vi "Test - Restartable.vi"() -> ()   [LabVIEW 2018]
uses:
  Ammeter.ctl
  <vilib>/DAQmx/read.llb/DAQmx Read (Analog 1D Wfm NChan NSamp).vi
  <vilib>/DAQmx/create/channels.llb/DAQmx Create Channel (AI-Voltage-Basic).vi
  <vilib>/DAQmx/create/channels.llb/DAQmx Create Channel (CI-Pulse Ticks).vi
  <vilib>/DAQmx/miscellaneous.llb/DAQmx Fill In Error Info.vi
panel:
  in  "?":enum32{"Monitor", "Calibration", "Future Use"}(tab)
  out "GPMDischarge":T1 caption="Dis GPM" format="%2.0f"
  out "GPMCase":T1 caption="Case GPM" format="%2.0f"
  out "PSI Case":T1 caption="Case PSI" format="%2.0f"
  out "PSI In":T1 caption="Inlet PSI" format="%2.0f"
  out "PSI Discharge":T1 caption="Dis PSI" format="%2.0f"
  out "Amps C":dbl format="%#.2g"
  out "Amps B":dbl format="%#.2g"
  out "Amps A":dbl format="%#.2g"
  out "VAC C":dbl caption="Vac" format="%#_3f"
  out "VAC B":dbl caption="Vac" format="%#_3f"
  out "VAC A":dbl caption="Vac" format="%#_3f"
  out "AC Hz":dbl caption="Hz" format="%#_3f"
  in  "Stop Button":bool
  in  "Loop Delay":u32=5
  out "Waveform Chart":waveform(dbl)[](graph)
  in  "Stop Button 2":bool
  in  "Boolean":bool
  in  "CaseGPM Offset":dbl format="%#_13g"
  in  "CaseGPM Scale":dbl=1.0 format="%#_13g"
  out "CaseGPM":dbl caption="Indicated"
  in  "DisGPM Offset":dbl format="%#_13g"
  in  "DisGPM Scale":dbl=1.0 format="%#_13g"
  out "DisGPM":dbl caption="Indicated"
  in  "CasePSI Offset":dbl format="%#_13g"
  in  "CasePSI Scale":dbl=200.0 format="%#_13g"
  out "CasePSI":dbl caption="Indicated"
  in  "InPSI Offset":dbl format="%#_13g"
  in  "InPSI Scale":dbl=100.0 format="%#_13g"
  out "InPSI Ind":dbl caption="Indicated"
  in  "DisPSI Offset":dbl format="%#_13g"
  in  "DisPSI Scale":dbl=1000.0 format="%#_13g"
  out "DisPSI Ind":dbl caption="Indicated"
  out "AC Freq Ind":dbl caption="Indicated"
  in  "AC Freq Offset":dbl=10.0 caption="Offset" format="%#_13g"
  in  "AC Freq Scale":dbl=100.0 caption="Scale" format="%#_13g"
  out "A VAC Ind":dbl caption="Indicated"
  in  "VAC Offset A":dbl caption="Offset" format="%#_13g"
  in  "VAC Scale A":dbl=50.0 caption="Scale" format="%#_13g"
  out "B VAC Ind":dbl caption="Indicated"
  in  "Amp Offset C":dbl format="%#_13g"
  in  "Amp Offset B":dbl format="%#_13g"
  in  "Amp Offset A":dbl format="%#_13g"
  in  "Amp Scale C":dbl=9.88 format="%#_13g"
  in  "Amp Scale B":dbl=9.88 format="%#_13g"
  in  "Amp Scale A":dbl=9.88 format="%#_13g"
  in  "VAC Scale B":dbl=50.0 caption="Scale" format="%#_13g"
  in  "VAC Offset B":dbl caption="Offset" format="%#_13g"
  in  "VAC Offset C":dbl caption="Offset" format="%#_13g"
  in  "VAC Scale C":dbl=50.0 caption="Scale" format="%#_13g"
  out "C VAC Ind":dbl caption="Indicated"
  out "A VAmp Ind":dbl caption="Indicated"
  out "B VAmp Ind":dbl caption="Indicated"
  out "C VAmp Ind":dbl caption="Indicated"
  out "error out":errorcluster
  # "AC Frequency"
  # "A Phase VAC"
  # "B Phase VAC"
  # "C Phase VAC"
  # "A Phase Amps"
  # "B Phase Amps"
  # "C Phase Amps"
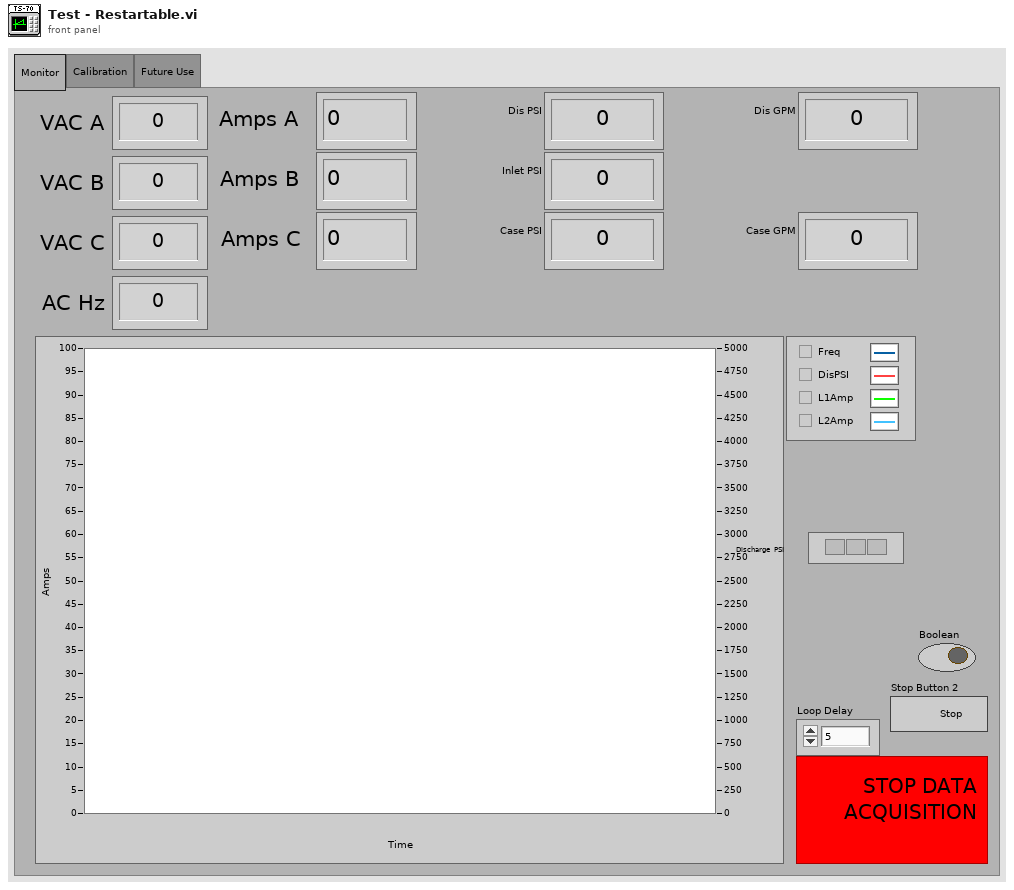
[diagram p1: front panel]
types:
  T1 = typedef "Ammeter.ctl" = dbl
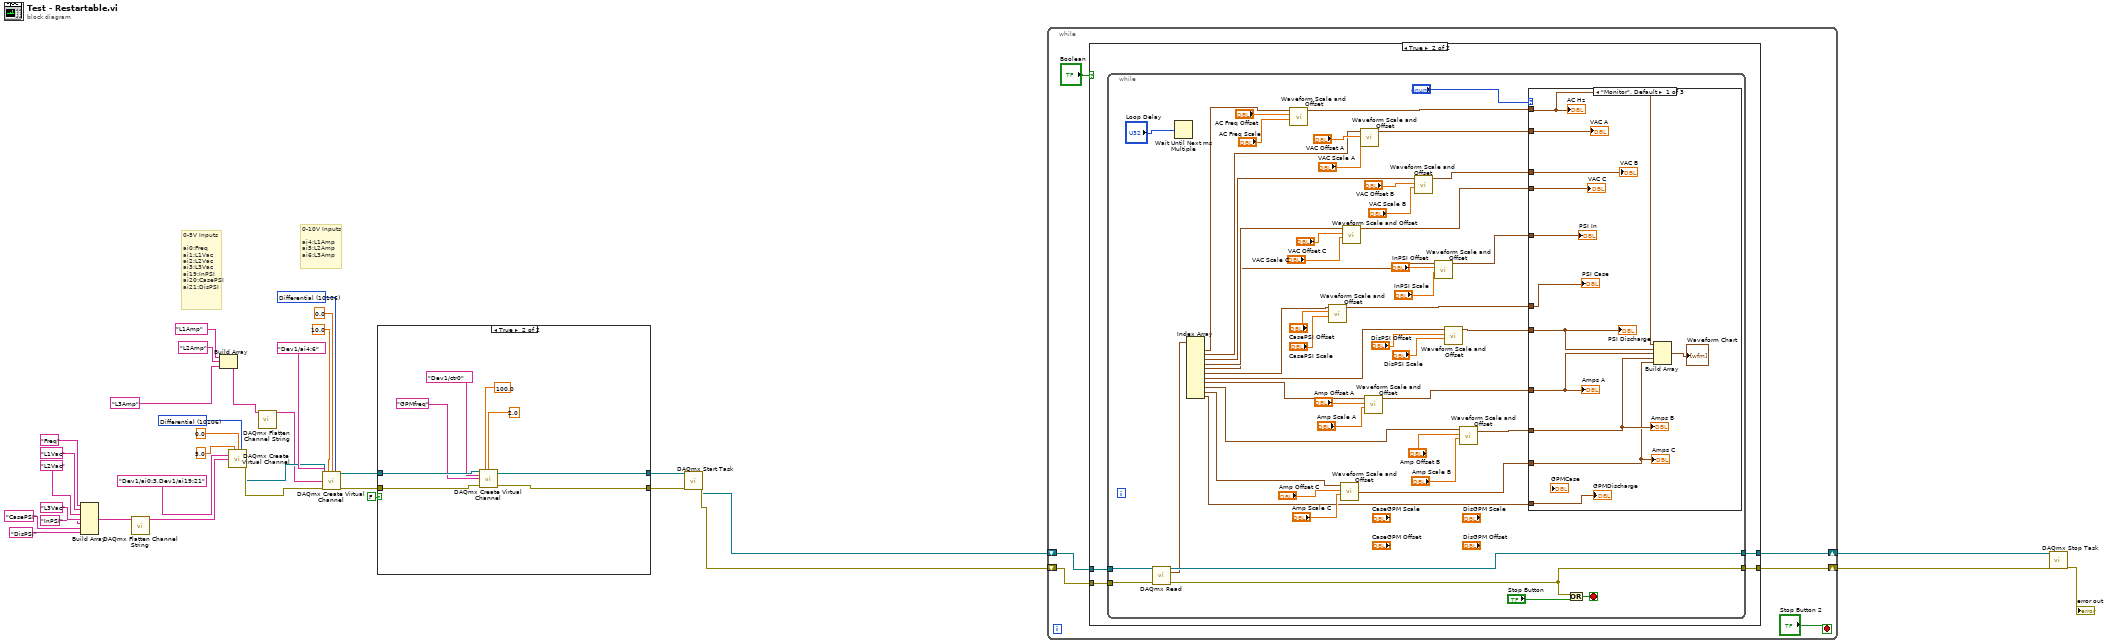
[diagram p0: block diagram]
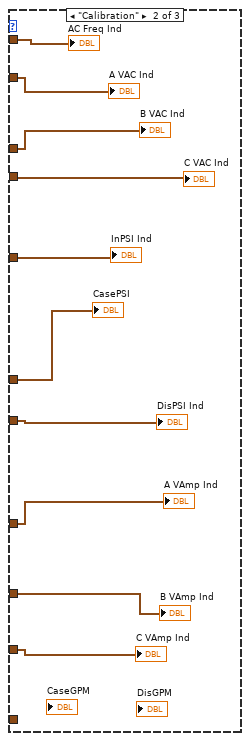
[diagram p4: hidden frame]
diagram:
  w28 = 10106 items=["default"=-1, "RSE"=10083, "NRSE"=10078, "Differential"=10106, "Pseudodifferential"=12529] ("input terminal configuration")
  w31 = 10106 items=["default"=-1, "RSE"=10083, "NRSE"=10078, "Differential"=10106, "Pseudodifferential"=12529] ("input terminal configuration")
  # "0-10V Inputs\n\nai4:L1Amp\nai5:L2Amp\nai6:L3Amp"
  # "0-5V Inputs\n\nai0:Freq\nai1:L1Vac\nai2:L2Vac\nai3:L3Vac\nai19:InPSI\nai20:CasePSI\nai21:DisPSI"
  n1 = Build Array("Freq", "L1Vac", "L2Vac", "L3Vac", "InPSI" ("element"), "CasePSI", "DisPSI") -> (w14:string[])
  n2 = call <vilib>:"DAQmx Flatten Channel String.vi"("names in"=w14) -> ("names out"=w13:string)  [unwired: 13 in, 1 out]
  n3 = Build Array("L1Amp", "L2Amp", "L3Amp") -> (w11:string[])
  n4 = call-poly <vilib>:"DAQmx Create Virtual Channel.vi"("maximum value"=5.0, "minimum value"=0.0, "input terminal configuration"=w31, "physical channels"=tag "Dev1/ai0:3,Dev1/ai19:21", "name to assign"=w13) -> ("task out"=w24:refnum<k21>, "error out"=w25:errorcluster)  [unwired: 9 in]
  n5 = call <vilib>:"DAQmx Flatten Channel String.vi"("names in"=w11) -> ("names out"=w7:string)  [unwired: 13 in, 1 out]
  n6 = call-poly <vilib>:"DAQmx Create Virtual Channel.vi"("task in"=w24, "maximum value"=10.0, "minimum value"=0.0, "input terminal configuration"=w28, "physical channels"=tag "Dev1/ai4:6", "name to assign"=w7, "error in"=w25) -> ("task out"=w5:refnum<k21>, "error out"=w3:errorcluster)  [unwired: 7 in]
  n7 = case shown="True" FALSE {
    tunnel: w5 -> [w36 w44]
    tunnel: [w36 w43] -> w4
    tunnel: w3 -> [w35 w42]
    tunnel: [w35 w41] -> w2
    frame False {
    }
    frame True {
      n8 = call-poly <vilib>:"DAQmx Create Virtual Channel.vi"("task in"=w44, "maximum value"=100.0, "minimum value"=2.0, "counter"=tag "Dev1/ctr0", "name to assign"="GPMfreq", "error in"=w42) -> ("task out"=w43:refnum<k21>, "error out"=w41:errorcluster)  [unwired: 8 in]
    }
  }
  n9 = call <vilib>:"DAQmx Start Task.vi"("task/channels in"=w4, "error in"=w2) -> ("task out"=w6:refnum<k21>, "error out"=w34:errorcluster)  [unwired: 12 in]
  n10 = while {
    shift-right: [w49] -> w23
    shift-left: w34 -> [w50]
    shift-right: [w48] -> w22
    shift-left: w6 -> [w47]
    stop <- "Stop Button 2" stop-if-true
    n11 = case shown="True" "Boolean" {
      tunnel: w50 -> [w51 w56]
      tunnel: [w51 w55] -> w49
      tunnel: [w52 w54] -> w48
      tunnel: w47 -> [w52 w53]
      frame False {
      }
      frame True {
        n12 = while {
          tunnel: w53 -> [w106]
          tunnel: w56 -> [w105]
          tunnel: [w101] -> w55
          tunnel: [w100] -> w54
          stop <- w102 stop-if-true
          n13 = call-poly <vilib>:"DAQmx Read.vi"("task/channels in"=w106, "error in"=w105) -> ("task out"=w100:refnum<k21>, "data"=w87:waveform(dbl)[], "error out"=w101:errorcluster)  [unwired: 11 in]
          n14 = Wait Until Next ms Multiple(millisecond multiple="Loop Delay") -> ()  [unwired: 1 out]
          n15 = Index Array(array=w87) -> (element #1=w72:waveform(dbl), element #2=w88:waveform(dbl), element #3=w82:waveform(dbl), element #4=w81:waveform(dbl), element #5=w64:waveform(dbl), element #6=w59:waveform(dbl), element #7=w68:waveform(dbl), element #8=w97:waveform(dbl), element #9=w92:waveform(dbl), element #10=w91:waveform(dbl), element #11=w57:waveform(dbl))  [unwired: 11 in]
          n16 = call <vilib>:"Waveform Scale and Offset.vi"("scale"="AC Freq Scale", "offset"="AC Freq Offset", "waveform in"=w72) -> ("waveform out"=w73:waveform(dbl))  [unwired: 7 in, 1 out]
          n17 = call <vilib>:"Waveform Scale and Offset.vi"("scale"="CasePSI Scale", "offset"="CasePSI Offset", "waveform in"=w59) -> ("waveform out"=w58:waveform(dbl))  [unwired: 7 in, 1 out]
          n18 = call <vilib>:"Waveform Scale and Offset.vi"("scale"="Amp Scale C", "offset"="Amp Offset C", "waveform in"=w91) -> ("waveform out"=w71:waveform(dbl))  [unwired: 7 in, 1 out]
          n19 = call <vilib>:"Waveform Scale and Offset.vi"("scale"="VAC Scale C", "offset"="VAC Offset C", "waveform in"=w81) -> ("waveform out"=w77:waveform(dbl))  [unwired: 7 in, 1 out]
          n20 = call <vilib>:"Waveform Scale and Offset.vi"("scale"="VAC Scale A", "offset"="VAC Offset A", "waveform in"=w88) -> ("waveform out"=w79:waveform(dbl))  [unwired: 7 in, 1 out]
          n21 = call <vilib>:"Waveform Scale and Offset.vi"("scale"="Amp Scale A", "offset"="Amp Offset A", "waveform in"=w97) -> ("waveform out"=w70:waveform(dbl))  [unwired: 7 in, 1 out]
          n22 = call <vilib>:"Waveform Scale and Offset.vi"("scale"="VAC Scale B", "offset"="VAC Offset B", "waveform in"=w82) -> ("waveform out"=w78:waveform(dbl))  [unwired: 7 in, 1 out]
          n23 = call <vilib>:"Waveform Scale and Offset.vi"("scale"="InPSI Scale", "offset"="InPSI Offset", "waveform in"=w64) -> ("waveform out"=w65:waveform(dbl))  [unwired: 7 in, 1 out]
          n24 = call <vilib>:"Waveform Scale and Offset.vi"("scale"="DisPSI Scale", "offset"="DisPSI Offset", "waveform in"=w68) -> ("waveform out"=w69:waveform(dbl))  [unwired: 7 in, 1 out]
          n25 = call <vilib>:"Waveform Scale and Offset.vi"("scale"="Amp Scale B", "offset"="Amp Offset B", "waveform in"=w92) -> ("waveform out"=w76:waveform(dbl))  [unwired: 7 in, 1 out]
          n26 = case shown="\"Monitor\", Default" "?" {
            tunnel: w79 -> [w118 w128 _]
            tunnel: w78 -> [w117 w126 _]
            tunnel: w77 -> [w116 w125 _]
            tunnel: w76 -> [w110 w124 _]
            tunnel: w71 -> [w109 w121 _]
            tunnel: w73 -> [w108 w127 _]
            tunnel: w70 -> [w115 w123 _]
            tunnel: w69 -> [w114 w122 _]
            tunnel: w65 -> [w112 w120 _]
            tunnel: w58 -> [w111 w119 _]
            tunnel: w57 -> [w107 _ _]
            frame "Monitor", Default {
              n27 = Build Array(w108, w114, w115, w110, w109) -> (→"Waveform Chart":waveform(dbl)[])
              "VAC A" <- w118
              "VAC B" <- w117
              "VAC C" <- w116
              "Amps B" <- w110
              "Amps C" <- w109
              "AC Hz" <- w108
              "Amps A" <- w115
              "PSI Discharge" <- w114
              "PSI In" <- w112
              "PSI Case" <- w111
              "GPMDischarge" <- w107
            }
            frame "Calibration" {
              "A VAC Ind" <- w128
              "B VAC Ind" <- w126
              "C VAC Ind" <- w125
              "A VAmp Ind" <- w123
              "B VAmp Ind" <- w124
              "C VAmp Ind" <- w121
              "AC Freq Ind" <- w127
              "DisPSI Ind" <- w122
              "InPSI Ind" <- w120
              "CasePSI" <- w119
            }
            frame "Future Use" {
            }
          }
          n28 = Or(x=w101, y="Stop Button") -> (x .or. y?=w102:bool)
        }
      }
    }
  }
  n29 = call <vilib>:"DAQmx Stop Task.vi"("task/channels in"=w22, "error in"=w23) -> ("error out"=→"error out":errorcluster)  [unwired: 12 in, 1 out]
